vi "FeatureAgglomeration.vi"(8 "error in":errorcluster) -> (0 "error out":errorcluster, 3 "out":refnum<class "FeatureAgglomeration.lvclass">)   [LabVIEW 2020]
doc: "Agglomerate features.\n\n Similar to AgglomerativeClustering, but recursively merges features\n instead of samples.\n\n Read more in the :ref:`User Guide <hierarchical_clustering>`.\n\n Parameters\n ----------\n n_clusters : int, default=2\n The number of clusters to find. It must be ``None`` if\n ``distance_threshold`` is not ``None``.\n\n affinity : str or callable, default='euclidean'\n Metric used to compute the linkage. Can be \"euclidean\", \"l1\", \"l2\",\n \"manhattan\", \"cosine\", or 'precomputed'.\n If linkage is \"ward\", only \"euclidean\" is accepted.\n\n memory : str or object with the joblib.Memory interface, default=None\n Used to cache the output of the computation of the tree.\n By default, no caching is done. If a string is given, it is the\n path to the caching directory.\n\n connectivity : array-like or callable, default=None\n Connectivity matrix. Defines for each feature the neighboring\n features following a given structure of the data.\n This can be a connectivity matrix itself or a callable that transforms\n the data into a connectivity matrix, such as derived from\n kneighbors_graph. Default is None, i.e, the\n hierarchical clustering algorithm is unstructured.\n\n compute_full_tree : 'auto' or bool, default='auto'\n Stop early the construction of the tree at n_clusters. This is useful\n to decrease computation time if the number of clusters is not small\n compared to the number of features. This option is useful only when\n specifying a connectivity matrix. Note also that when varying the\n number of clusters and using caching, it may be advantageous to compute\n the full tree. It must be ``True`` if ``distance_threshold`` is not\n ``None``. By default `compute_full_tree` is \"auto\", which is equivalent\n to `True` when `distance_threshold` is not `None` or that `n_clusters`\n is inferior to the maximum between 100 or `0.02 * n_samples`.\n Otherwise, \"auto\" is equivalent to `False`.\n\n linkage : {'ward', 'complete', 'average', 'single'}, default='ward'\n Which linkage criterion to use. The linkage criterion determines which\n distance to use between sets of features. The algorithm will merge\n the pairs of cluster that minimize this criterion.\n\n - ward minimizes the variance of the clusters being merged.\n - average uses the average of the distances of each feature of\n the two sets.\n - complete or maximum linkage uses the maximum distances between\n all features of the two sets.\n - single uses the minimum of the distances between all features\n of the two sets.\n\n pooling_func : callable, default=np.mean\n This combines the values of agglomerated features into a single\n value, and should accept an array of shape [M, N] and the keyword\n argument `axis=1`, and reduce it to an array of size [M].\n\n distance_threshold : float, default=None\n The linkage distance threshold above which, clusters will not be\n merged. If not ``None``, ``n_clusters`` must be ``None`` and\n ``compute_full_tree`` must be ``True``.\n\n .. versionadded:: 0.21\n\n compute_distances : bool, default=False\n Computes distances between clusters even if `distance_threshold` is not\n used. This can be used to make dendrogram visualization, but introduces\n a computational and memory overhead.\n\n .. versionadded:: 0.24\n\n Attributes\n ----------\n n_clusters_ : int\n The number of clusters found by the algorithm. If\n ``distance_threshold=None``, it will be equal to the given\n ``n_clusters``.\n\n labels_ : array-like of (n_features,)\n cluster labels for each feature.\n\n n_leaves_ : int\n Number of leaves in the hierarchical tree.\n\n n_connected_components_ : int\n The estimated number of connected components in the graph.\n\n .. versionadded:: 0.21\n ``n_connected_components_`` was added to replace ``n_components_``.\n\n children_ : array-like of shape (n_nodes-1, 2)\n The children of each non-leaf node. Values less than `n_features`\n correspond to leaves of the tree which are the original samples.\n A node `i` greater than or equal to `n_features` is a non-leaf\n node and has children `children_[i - n_features]`. Alternatively\n at the i-th iteration, children[i][0] and children[i][1]\n are merged to form node `n_features + i`\n\n distances_ : array-like of shape (n_nodes-1,)\n Distances between nodes in the corresponding place in `children_`.\n Only computed if `distance_threshold` is used or `compute_distances`\n is set to `True`.\n\n \nAvailable methods:\nGet Attributes\nGet Params\nSet Params"
uses:
  FeatureAgglomeration.lvclass
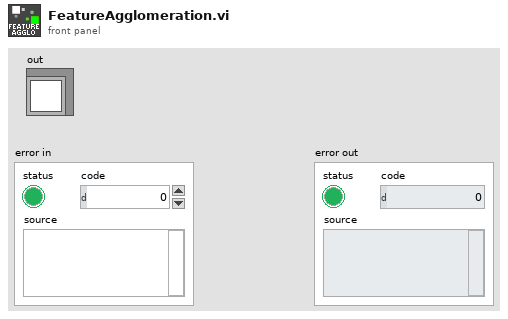
[diagram p1: front panel]
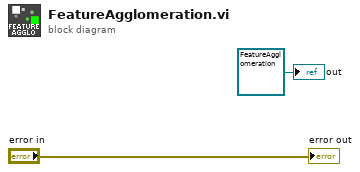
[diagram p0: block diagram]
diagram:
  "out" <- refnum<class "FeatureAgglomeration.lvclass"> refnum ("model")
  "error out" <- "error in"
